vi "setTimeStamp.vi"(8 "error in (no error)":errorcluster, 10 "timeStamp":string, 11 "ScriptListCompiler in":refnum<class "ScriptListCompiler.lvclass">) -> (0 "error out":errorcluster, 3 "ScriptListCompiler out":refnum<class "ScriptListCompiler.lvclass">)   [LabVIEW 2009, in "Compiler.lvlib" / "ScriptListCompiler.lvclass"]
uses:
  ScriptListCompiler.lvclass
  ScriptListCompiler.lvclass/ScriptListCompiler.ctl
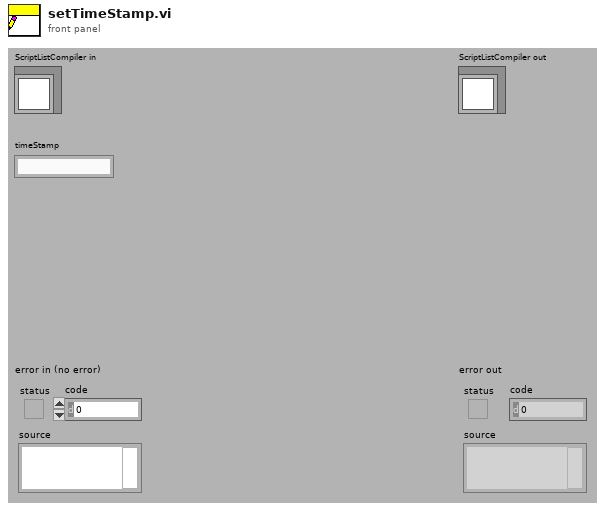
[diagram p1: front panel]
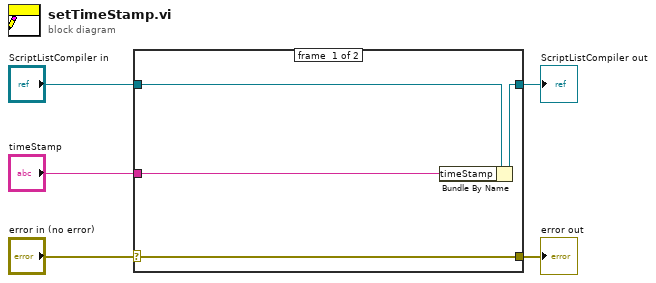
[diagram p0: block diagram]
diagram:
  n1 = case shown="No Error" "error in (no error)" {
    selector: "error in (no error)" -> [w9 w10]
    tunnel: [w9 w10] -> w4
    tunnel: [w7 w11] -> w2
    tunnel: "ScriptListCompiler in" -> [w8 w11]
    tunnel: "timeStamp" -> [w6 _]
    frame #0 {
      n2 = Bundle By Name(cluster=w8, "timeStamp"=w6) -> (w7:refnum<class "ScriptListCompiler.lvclass">)
    }
    frame #1 {
    }
  }
  "error out" <- w4
  "ScriptListCompiler out" <- w2
